vi "Get BlackLevelRange.vi"(8 "error in (no error)":errorcluster, 11 "TLCamera reference in":refnum<k24>) -> (0 "error out":errorcluster, 1 "Maximum":u32, 2 "Minimum":u32, 3 "TLCamera reference out":refnum<k24>)   [LabVIEW 2015]
uses:
  C:/code/Host/Installer/Scientific Camera Interfaces/LabVIEW/32_bit/Library_X86/Thorlabs.TSI.TLCameraInterfaces.dll
  code/Host/Installer/Scientific Camera Interfaces/LabVIEW/32_bit/Library_X86/Thorlabs.TSI.TLCameraInterfaces.dll
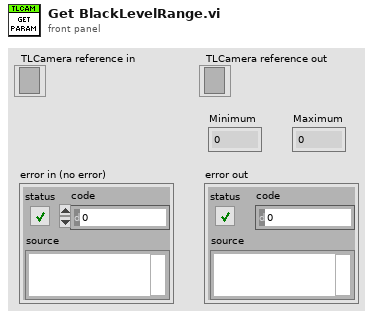
[diagram p1: front panel]
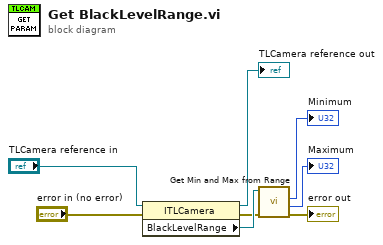
[diagram p0: block diagram]
diagram:
  n1 = property class="ITLCamera"(reference="TLCamera reference in", error in="error in (no error)") -> (reference out=→"TLCamera reference out":refnum<k24>, error out=w4:errorcluster, "BlackLevelRange"=w5:refnum<k24>)
  n2 = call "Get Min and Max from Range.vi"("error in (no error)"=w4, "BinXRange"=w5) -> ("error out"=→"error out":errorcluster, "Maximum"=→"Maximum":u32, "Minimum"=→"Minimum":u32)  [unwired: 7 in]
